vi "pshtr.vi"(0 "Boolean":bool, 2 "VISA resource name":refnum<visa-resource-name>) -> ()   [LabVIEW 2015]
panel:
  out "millisecond timer value 2":u32
  out "error out":errorcluster
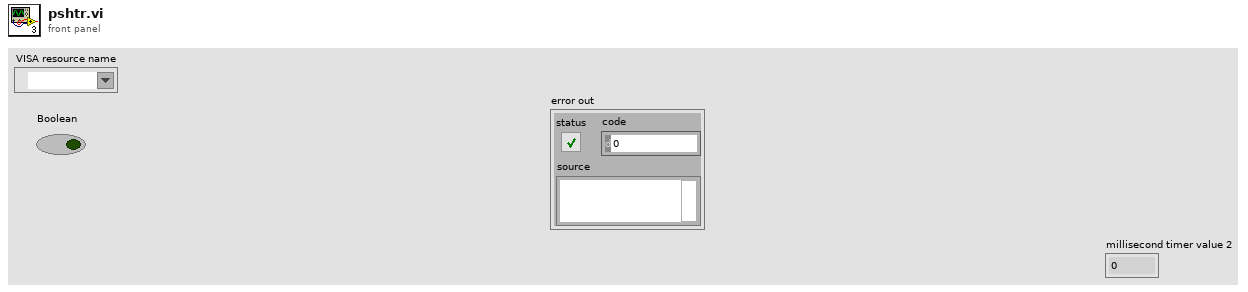
[diagram p1: front panel]
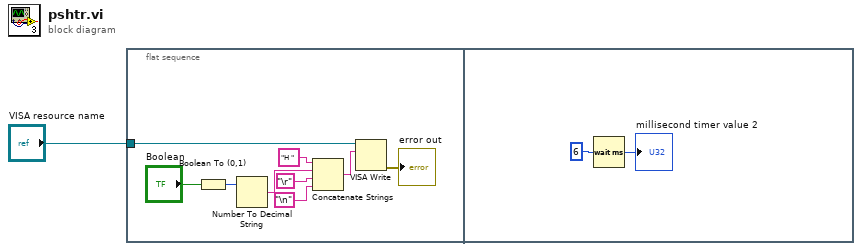
[diagram p0: block diagram]
diagram:
  n1 = flat-sequence {
    tunnel: "VISA resource name" -> [w2]
    frame #0 {
      n2 = Boolean To (0,1)(Boolean="Boolean") -> (0, 1=w9:i16)
      n3 = Number To Decimal String(number=w9) -> (decimal integer string=w7:string)  [unwired: 1 in]
      n4 = Concatenate Strings("H " ("string"), w7, "\r", "\n") -> (w6:string)
      n5 = VISA Write(VISA resource name=w2, write buffer=w6) -> (error out=→"error out":errorcluster)  [unwired: 1 in, 2 out]
    }
    frame #1 {
      n6 = Wait (ms)(milliseconds to wait=u32 6) -> (millisecond timer value=→"millisecond timer value 2":u32)
    }
  }
